vi "Online Filtering.vi"() -> ()   [LabVIEW 2023]
doc: "Uses the IIR Cascade Filter VI to perform online filtering without having to compensate for the initial transient after the first block of data is filtered.\n\nThis example repeatedly generates a noisy sine wave and filters it using two different methods. \n\nThe first method uses the memory mechanism of the IIR Cascade Filter VI to retain state information about previous inputs and outputs of the filter in order to eliminate the transient. \n\nThe second method uses no memory mechanism causing the IIR Cascade Filter VI to assume zero initial conditions each time the VI is called. The result is that on each iteration this method produces a transient rather than the filtered signal."
uses:
  <vilib>/Analysis/3filter.llb/Filter Passband Type.ctl
  <vilib>/Analysis/baseanly.llb/IIR Cascade Filter (DBL).vi
  <vilib>/Analysis/NI_AALBase.lvlib
panel:
  out "Filtered Waveform Graph":dbl[][](graph)
  in  "# points":i32=100
  in  "Stop":bool
  # "Overview: Demonstrates the use of the IIR Cascade Filter VI to perform online filtering.\nRequirements: LabVIEW Full Development System\nInstructions:\n1. Run the VI.\n2. Observe that the single mode trace always has a transient at the beginning of the waveform in the Filtered Waveform Graph.\n3. Click Stop to stop the VI."
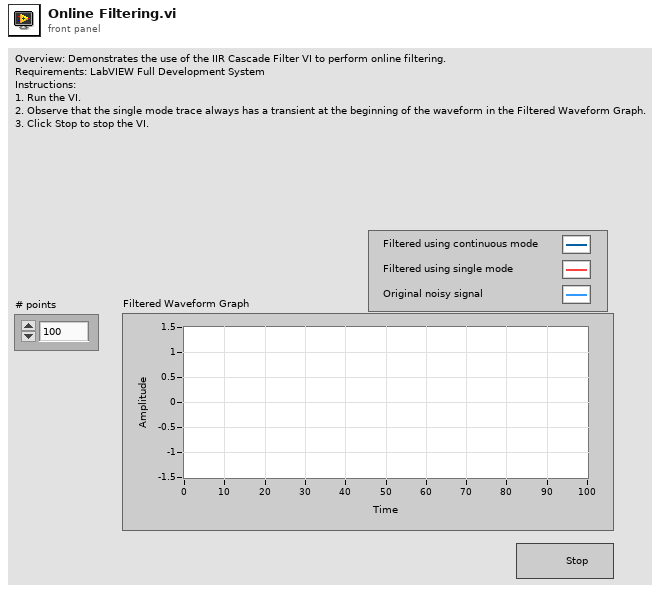
[diagram p1: front panel]
types:
  T1 = typedef "NI_AALBase.lvlib/Filter Passband Type.ctl" = enum32{"Lowpass", "Highpass", "Bandpass", "Bandstop"}
  T2 = cluster{"filter structure":enum32{"IIR 2nd Order", "IIR 4th Order"}, "Reverse Coefficients":dbl[], "Forward Coefficients":dbl[]}
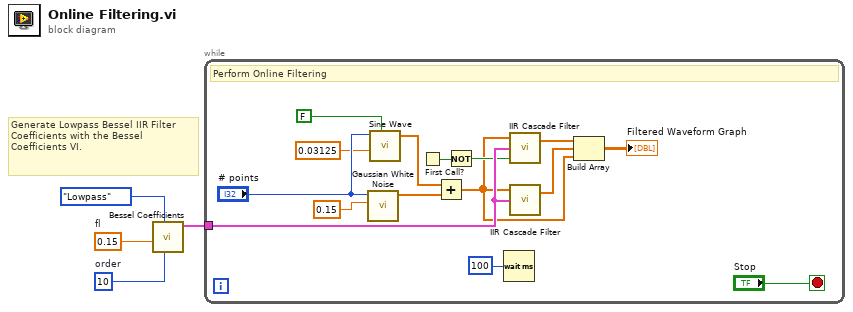
[diagram p0: block diagram]
diagram:
  w1 = 10  # order
  w2 = 0.15  # fl
  # "Generate Lowpass Bessel IIR Filter \nCoefficients with the Bessel Coefficients VI."
  n1 = call <vilib>:"Bessel Coefficients.vi"("order"=w1, "filter type"=Filter_Passband_Type."Lowpass", "low cutoff freq: fl"=w2) -> ("IIR Filter Cluster"=w4:T2)  [unwired: 7 in, 1 out]
  n2 = while {
    tunnel: w4 -> [w16]
    stop <- "Stop" stop-if-true
    # "Perform Online Filtering"
    n3 = call <vilib>:"Gaussian White Noise.vi"("standard deviation"=0.15, "samples"="# points") -> ("Gaussian noise pattern"=w19:dbl[])  [unwired: 8 in, 1 out]
    n4 = call <vilib>:"Sine Wave.vi"("samples"="# points", "frequency"=0.03125, "reset phase"=FALSE) -> ("sine wave"=w15:dbl[])  [unwired: 2 in, 2 out]
    n5 = First Call?() -> (First Call?: T/F=w12:bool)
    n6 = Add(x=w15, y=w19) -> (x+y=w7:dbl[])
    n7 = Not(x=w12) -> (.not. x?=w11:bool)
    n8 = Wait (ms)(milliseconds to wait=u32 100) -> ()  [unwired: 1 out]
    n9 = call-poly <vilib>:"IIR Cascade Filter.vi"("init/cont (init:F)"=w11, "IIR Filter Cluster"=w16, "X"=w7) -> ("Filtered X"=w10:dbl[])  [unwired: 1 out]
    n10 = call-poly <vilib>:"IIR Cascade Filter.vi"("IIR Filter Cluster"=w16, "X"=w7) -> ("Filtered X"=w9:dbl[])  [unwired: 1 in, 1 out]
    n11 = Build Array(w10, w9, w7) -> (→"Filtered Waveform Graph":dbl[][])
  }
